vi "GetSlaveControlReferences.vi"(8 "error in (no error)":errorcluster, 11 "VI in":refnum<vi>) -> (0 "error out":errorcluster, 2 "Control References":T1, 3 "VI out":refnum<vi>)   [LabVIEW 2018]
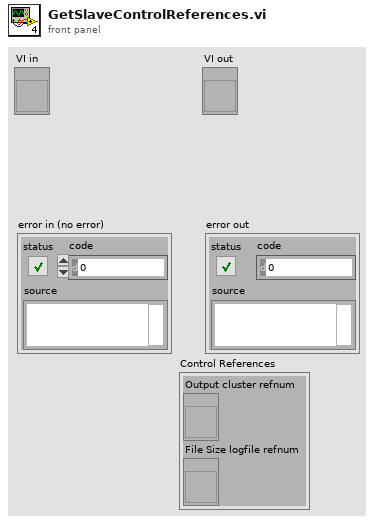
[diagram p1: front panel]
types:
  T1 = cluster{"Output cluster refnum":refnum<vi>, "File Size logfile refnum":refnum<vi>}
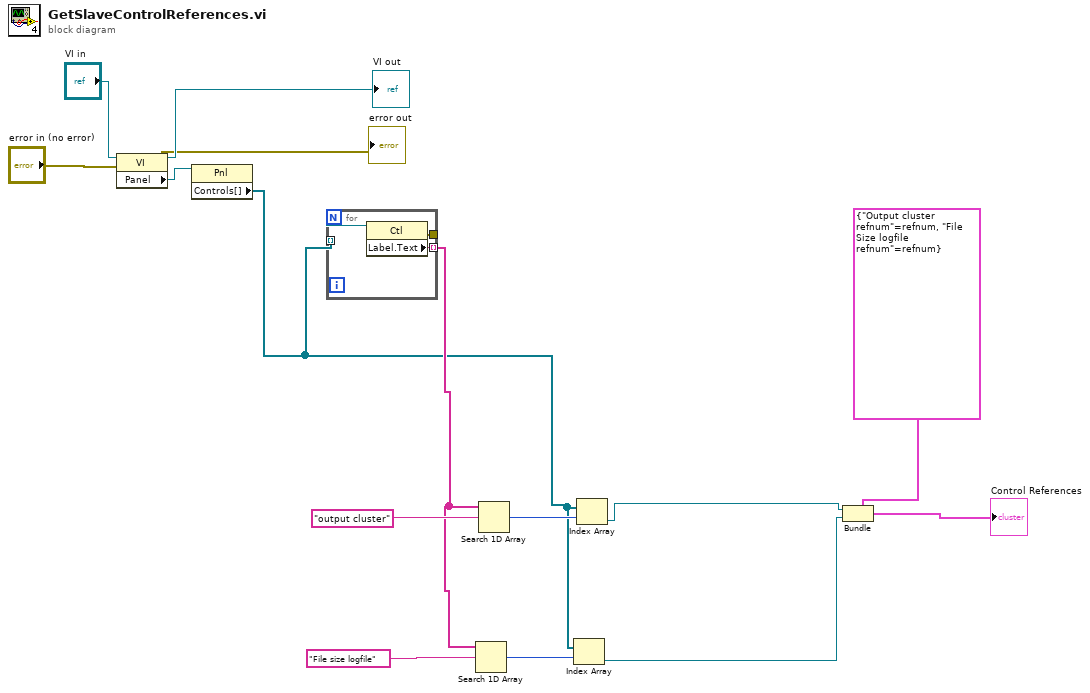
[diagram p0: block diagram]
diagram:
  n1 = property class="VI"(reference="VI in", error in="error in (no error)") -> (reference out=→"VI out":refnum<vi>, error out=→"error out":errorcluster, "Panel"=w11:refnum<vi>)
  n2 = property class="Pnl"(reference=w11) -> ("Controls[]"=w4:refnum<vi>[])  [unwired: 1 in, 2 out]
  n3 = for {
    tunnel: w4 -> [w18] mode=indexing
    tunnel: [w17] -> w5 mode=indexing
    tunnel: [w16] -> _
    n4 = property class="Ctl"(reference=w18) -> (error out=w16:errorcluster, "Label.Text"=w17:string)  [unwired: 1 in, 1 out]
  }
  n5 = Search 1D Array(1D array=w5, element="File size logfile") -> (index of element=w7:i32)  [unwired: 1 in]
  n6 = Search 1D Array(1D array=w5, element="output cluster") -> (index of element=w10:i32)  [unwired: 1 in]
  n7 = Index Array(array=w4, index=w7) -> (element=w2:refnum<vi>)
  n8 = Index Array(array=w4, index=w10) -> (element=w3:refnum<vi>)
  n9 = Bundle(cluster=T1 {"Output cluster refnum"=refnum, "File Size logfile refnum"=refnum}, "Output cluster refnum"=w3, "File Size logfile refnum"=w2) -> (→"Control References":T1)
